vi "Cryostation.GetAlltoStatusString.vi"(8 "error in (no error)":errorcluster, 11 "instrument.Cryostation in":refnum<class "instrument.Cryostation.lvclass">) -> (0 "error out":errorcluster, 2 "status string":string, 3 "instrument.Cryostation out":refnum<class "instrument.Cryostation.lvclass">)   [LabVIEW 2019, in "instrument.Cryostation.lvclass"]
uses:
  instrument.Cryostation.lvclass
  instrument.Cryostation.lvclass/instrument.Cryostation.ctl
  <vilib>/regexp/Match Regular Expression.xnode
  <vilib>/Utility/Data Type/NI_Data Type.lvlib
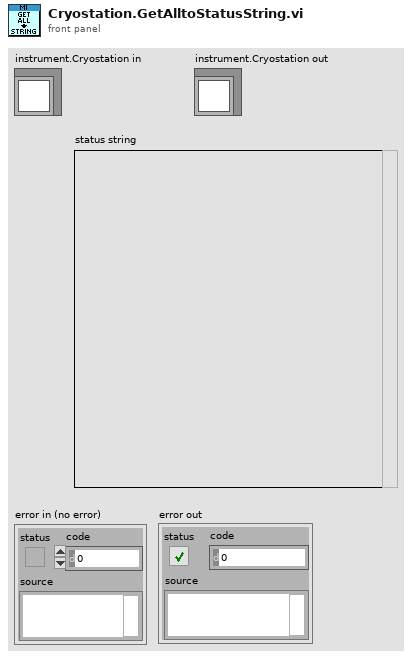
[diagram p1: front panel]
types:
  T1 = typedef "instrument.Cryostation.lvclass/Cryostation.getAll--cluster.ctl" = cluster{"Chamber Pressure (mTorr)":dbl, "Compressor Return Pressure (MPa)":dbl, "Compressor Supply Pressure (MPa)":dbl, "Compressor Speed (Hz)":dbl, "Cold Head Speed (Hz)":dbl, "Platform Heater Power (W)":dbl, "Platform Stability (K)":dbl, "Platform Temperature (K)":dbl, "Stage 1 Heater Power (W)":dbl, "Stage 1 Temperature (K)":dbl, "Stage 2 Heater Power (W)":dbl, "Stage 2 Temperature (K)":dbl, "Sample Stability (K)":dbl, "Sample Temperature (K)":dbl, "Temperature Set Point (K)":dbl, "User Stability (K)":dbl, "User Temperature (K)":dbl, "User Temperature Set Point (K)":dbl, "Alarm State":string, "Compressor Run State":string, "Case Valve State":string, "Idle State":string, "Nitrogen State":string, "Vent Valve State":string}
  T2 = typedef "NI_Data Type.lvlib/Data Type.ctl" = enum8{"Invalid Type", "Void", "I8", "I16", "I32", "I64", "U8", "U16", "U32", "U64", "Single Float", "Double Float", "Extended Float", "Single Complex", "Double Complex", "Extended Complex", "Enum U8", "Enum U16", "Enum U32", "Enum U64", "Single Float With Unit", "Double Float With Unit", "Extended Float With Unit", "Single Complex with Unit", "Double Complex with Unit", "Extended Complex with Unit", "Boolean", "String", "Path", "Picture", "Tag", "Array", "Cluster", "Variant", "LV Variant", "Waveform", "Timestamp", "Digital Waveform", "Digital Data", "ExpressData", "Refnum", "External Data", "VI", "Poly VI", "LabVIEW Class Instance", "Fixed Point", "Set Collection", "Map Collection"}
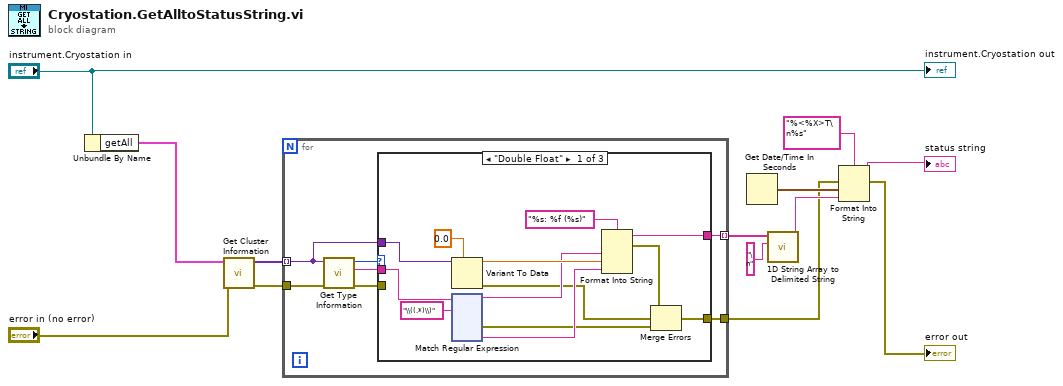
[diagram p0: block diagram]
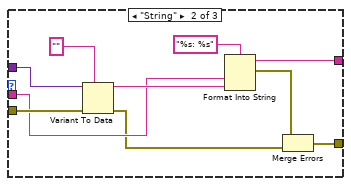
[diagram p2: hidden frame]
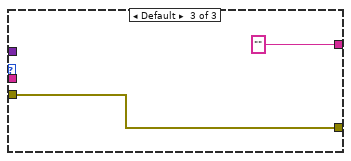
[diagram p3: hidden frame]
diagram:
  n1 = Unbundle By Name("instrument.Cryostation in") -> ("getAll"=w2:T1)
  n2 = call <vilib>:"Get Cluster Information.vi"("error in (no error)"="error in (no error)", "variant"=w2) -> ("error out"=w12:errorcluster, "cluster elements"=w13:variant[])  [unwired: 8 in]
  n3 = for {
    tunnel: w13 -> [w17] mode=indexing
    tunnel: w12 -> [w19]
    tunnel: [w15] -> w11 mode=indexing
    tunnel: [w14] -> w4
    n4 = call <vilib>:"Get Type Information.vi"("error in (no error)"=w19, "variant"=w17) -> ("error out"=w18:errorcluster, "name"=w16:string, "type"=w20:T2)  [unwired: 5 in, 2 out]
    n5 = case shown="\"Double Float\"" w20 {
      tunnel: w18 -> [_ w159 w160]
      tunnel: w17 -> [w32 w158 _]
      tunnel: w16 -> [w25 w153 _]
      tunnel: [w29 w155 ""] -> w15
      tunnel: [w21 w152 w160] -> w14
      frame "Double Float" {
        n6 = Variant To Data(type=0.0, Variant=w32) -> (data=w30:dbl, error out=w23:errorcluster)  [unwired: 1 in]
        n7 = xnode "Match Regular Expression"("input string"=w25, "regular expression"="\\((.*)\\)") -> ("before match"=w27:string, "error out"=w22:errorcluster, "submatch 1"=w28:string)  [unwired: 4 in, 3 out]
        n8 = Format Into String(format string="%s: %f (%s)", w27, w30, w28) -> (resulting string=w29:string, error out=w24:errorcluster)  [unwired: 2 in]
        n9 = Merge Errors(w24, w23, w22) -> (w21:errorcluster)
      }
      frame "String" {
        n10 = Variant To Data(error in=w159, type="" ("format string"), Variant=w158) -> (data=w156:string, error out=w150:errorcluster)
        n11 = Format Into String(format string="%s: %s", w153, w156) -> (resulting string=w155:string, error out=w151:errorcluster)  [unwired: 2 in]
        n12 = Merge Errors(w151, w150) -> (w152:errorcluster)
      }
      frame Default {
      }
    }
  }
  n13 = Get Date/Time In Seconds() -> (seconds since 1Jan1904=w7:timestamp)
  n14 = call <vilib>:"1D String Array to Delimited String.vi"("delimiter"="\n", "string array"=w11) -> ("delimited string"=w6:string)  [unwired: 9 in]
  n15 = Format Into String(format string="%<%X>T\n%s", error in=w4, w7, w6) -> (resulting string=→"status string":string, error out=→"error out":errorcluster)  [unwired: 1 in]
  "instrument.Cryostation out" <- "instrument.Cryostation in"
